vi "FGVGenerate.vi"() -> ()   [LabVIEW 2014]
panel:
  out "GenerateCnt":i32
  in  "stop":bool
  out "32bit integer":i32
  # "Generate"
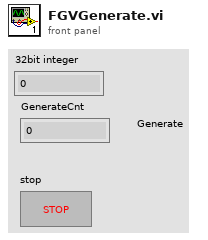
[diagram p1: front panel]
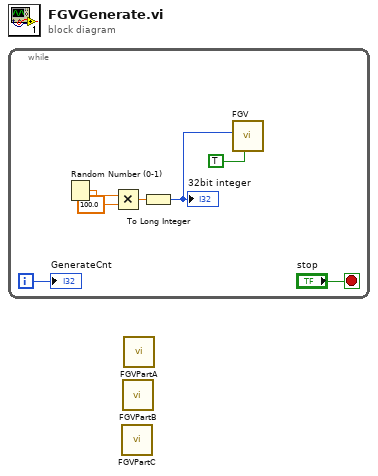
[diagram p0: block diagram]
diagram:
  n1 = while {
    i -> [w1]
    stop <- "stop" stop-if-true
    n2 = Random Number (0-1)() -> (number: 0 to 1=w7:dbl)
    n3 = Multiply(x=w7, y=100.0) -> (x*y=w5:dbl)
    n4 = To Long Integer(number=w5) -> (32bit integer=w4:i32)
    "32bit integer" <- w4
    n5 = call "FGV.vi"("Write"=TRUE, "Numeric"=w4) -> ()  [unwired: 9 in, 1 out]
    "GenerateCnt" <- w1
  }
  n6 = call "FGVPartC.vi"() -> ()  [unwired: 12 in]
  n7 = call "FGVPartB.vi"() -> ()  [unwired: 12 in]
  n8 = call "FGVPartA.vi"() -> ()  [unwired: 12 in]
